vi "Find Named XML Item.vi"(8 "error in":errorcluster, 10 "Name":string, 11 "Parent Node":refnum<k20>) -> (0 "error out":errorcluster, 1 "found?":bool, 2 "Named Node":refnum<k20>, 3 "Parent Node out":refnum<k20>)   [LabVIEW 2020, in "Template Tool.lvlib"]
uses:
  Template Tool.lvlib
  <vilib>/xml/NI_XML.lvlib
  <vilib>/xml/Close Reference(Node).vi
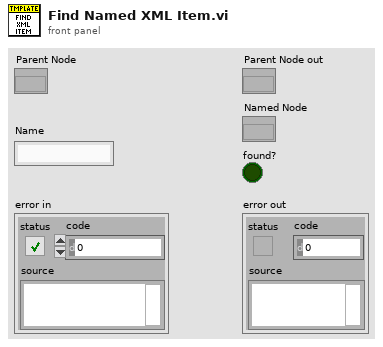
[diagram p1: front panel]
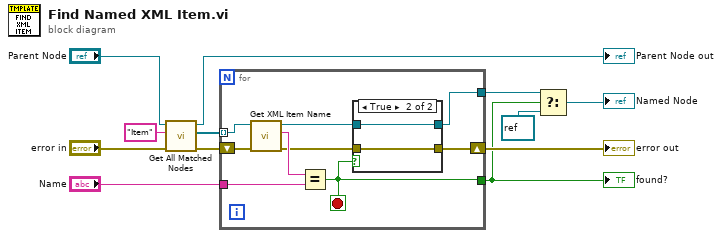
[diagram p0: block diagram]
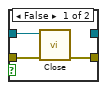
[diagram p2: hidden frame]
diagram:
  n1 = call <vilib>:"Get All Matched Nodes.vi"("error in (no error)"="error in", "XPath expression"="Item", "node in"="Parent Node") -> ("error out"=w10:errorcluster, "node result array"=w9:refnum<k20>[], "node out"=→"Parent Node out":refnum<k20>)  [unwired: 6 in]
  n2 = for {
    shift-right: [w15] -> w4
    shift-left: w10 -> [w21]
    tunnel: w9 -> [w20] mode=indexing
    tunnel: "Name" -> [w18]
    tunnel: [w16] -> w3
    tunnel: [w13] -> w7
    stop <- w16 stop-if-true
    n3 = call "Get XML Item Name.vi"("error in"=w21, "Node"=w20) -> ("error out"=w17:errorcluster, "Name"=w19:string, "Node out"=w14:refnum<k20>)  [unwired: 7 in]
    n4 = Equal?(x=w19, y=w18) -> (x = y?=w16:bool)
    n5 = case shown="True" w16 {
      tunnel: w17 -> [w24 w26]
      tunnel: [w23 w26] -> w15
      tunnel: w14 -> [w22 w25]
      tunnel: [_ w25] -> w13
      frame False {
        n6 = call-poly <vilib>:"Close.vi"("error in (no error)"=w24, "node"=w22) -> ("error out"=w23:errorcluster)  [unwired: 7 in]
      }
      frame True {
      }
    }
  }
  "error out" <- w4
  "found?" <- w3
  n7 = Select(t=w7, s=w3, f=refnum<k20> refnum) -> (s? t:f=→"Named Node":refnum<k20>)
